vi "测验程序2.vi"() -> ()   [LabVIEW 2017]
uses:
  <vilib>/userdefined/High Color/IMAQdx.ctl
  <vilib>/Platform/TimedLoop/XDataNode/timing_clust.ctl
  <vilib>/Platform/TimedLoop/XDataNode/nitl_modes.ctl
  <vilib>/Platform/TimedLoop/XDataNode/wakeup.ctl
  <vilib>/myRIO/Common/Instrument Driver Framework/myRIO v1.0/UART/vis/myRIO v1.0 Close UART.vi
  <vilib>/FPGAPlugInAG/myRIO-1900/niLvFpga_Open_myRIO-1900.vi
  <vilib>/rvi/interface/common/dynamic/niFpgaDynamicAddResources.vi
  <vilib>/myRIO/Common/Instrument Driver Framework/Utilities/vis/FPGA Ref Manager.vi
  <vilib>/Utility/error.llb/Error Cluster From Error Code.vi
  <vilib>/myRIO/Common/Instrument Driver Framework/Utilities/vis/Ref Counter.vi
  <vilib>/rvi/errors/niLvFpgaAdjustHostInterfaceError.vi
  <vilib>/FPGAPlugInAG/Dynamic/niLvFpga_Close_Dynamic.vi
  <vilib>/myRIO/Common/Instrument Driver Framework/myRIO v1.0/myRIO v1.0 Reset FPGA.vi
  <vilib>/myRIO/Common/Instrument Driver Framework/myRIO v1.0/IRQ/vis/myRIO v1.0 IRQ Info FGV.vi
  <vilib>/myRIO/Common/Instrument Driver Framework/myRIO v1.0/IRQ/vis/myRIO v1.0 Timer IRQ Info FGV.vi
  <vilib>/myRIO/Common/Instrument Driver Framework/myRIO v1.0/IRQ/vis/myRIO v1.0 ISR Agent.vi
  <vilib>/Platform/TimedLoop/XDataNode/XDataNode.xnode
  <vilib>/rvi/interface/nirviOpenFPGA/nirviOpenFPGA.xnode
  <vilib>/rvi/interface/nirviReadWriteControl/nirviReadWriteControl.xnode
  <vilib>/rvi/interface/nirviCloseFPGA/nirviCloseFPGA.xnode
  <vilib>/Platform/TimedLoop/XDataNode/XDNodeRunTimeDep.lvlib
  <vilib>/myRIO/Instrument Drivers/Utilities/Utilities.lvlib
  NiFpgaLv.dll
  <vilib>/rvi/interface/Simulation/niFpgaSimulationCallBeginRW.vi
  <vilib>/vision/driver/NI_Vision_Acquisition_Software.lvlib
  <vilib>/vision/NI_Vision_Development_Module.lvlib
panel:
  in  "停止":bool
  out "Image Out":T1(plugin-control)
  out "数量":i32[](array[numeric])
  out "大小":dbl[](array[numeric])
  in  "保留图像？":bool
  in  "停止 2":bool
  out "货物类型":dbl
  in  "初始步态":u16
  in  "长度":i32=20000
  in  "开始":bool
  in  "思币得":i32=60
  out "QTI":bool
  out "当前步态":u16
  out "超声波":u32[](array[numeric])
  # "4小蓝"
  # "3小红"
  # "2大蓝"
  # "100000"
  # "1大红"
  # "70000"
  # "0异常"
  # "14600夹取高度"
  # "700夹住"
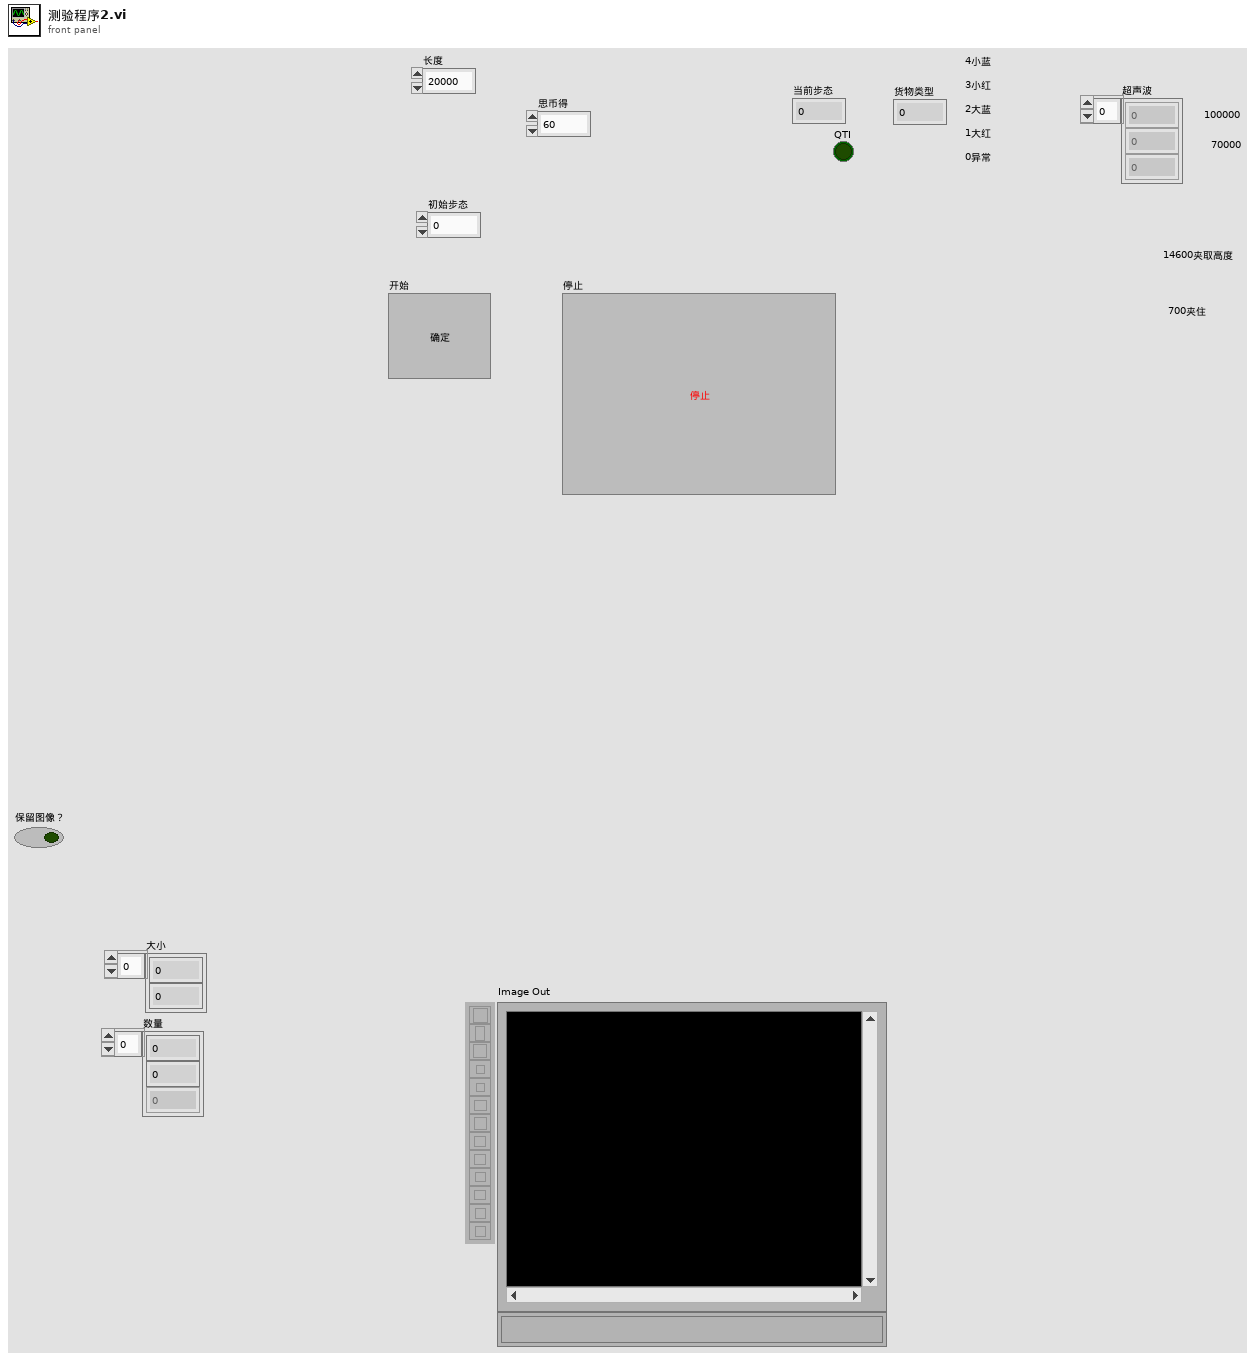
[diagram p1: front panel]
types:
  T1 = typedef "IMAQ Image.ctl" = refnum<image>
  T2 = typedef "IMAQdx.ctl" = refnum<k21>
  T3 = typedef "XDNodeRunTimeDep.lvlib/timing_clust.ctl" = cluster{"Expected End [f-1]":u64, "Actual End [f-1]":u64, "Finished Late? [f-1]":bool, "Expected End [i-1]":u64, "Actual End [i-1]":u64, "Finished Late? [i-1]":bool, "Expected Start [i]":u64, "Actual Start [i]":u64, "Expected Start [f]":u64, "Actual Start [f]":u64, "Source Name":string, "Structure Name":string, "Period":i64, "Deadline":i64, "Offset":i64, "Start":i64, "Priority":i32, "Timeout":i32, "Mode":T4, "Wakeup Reason":T5, "Error":errorcluster, "Source Type":string, "Secondary Source Type":string, "Global End Time":u64, "Global Start Time":u64, "Frame Duration":u64, "Iteration Duration":u64, "Assigned CPU":i32, "I/O Scan Engine Mode":u32}
  T4 = typedef "XDNodeRunTimeDep.lvlib/nitl_modes.ctl" = enum32{"No Change", "Process missed periods, maintain original phase", "Discard missed periods, maintain original phase", "Process missed periods, ignore original phase", "Discard missed periods, ignore original phase"}
  T5 = typedef "XDNodeRunTimeDep.lvlib/wakeup.ctl" = enum32{"Normal", "Aborted", "Asynchronous wakeup", "Timing source error", "Timed loop error", "Timeout"}
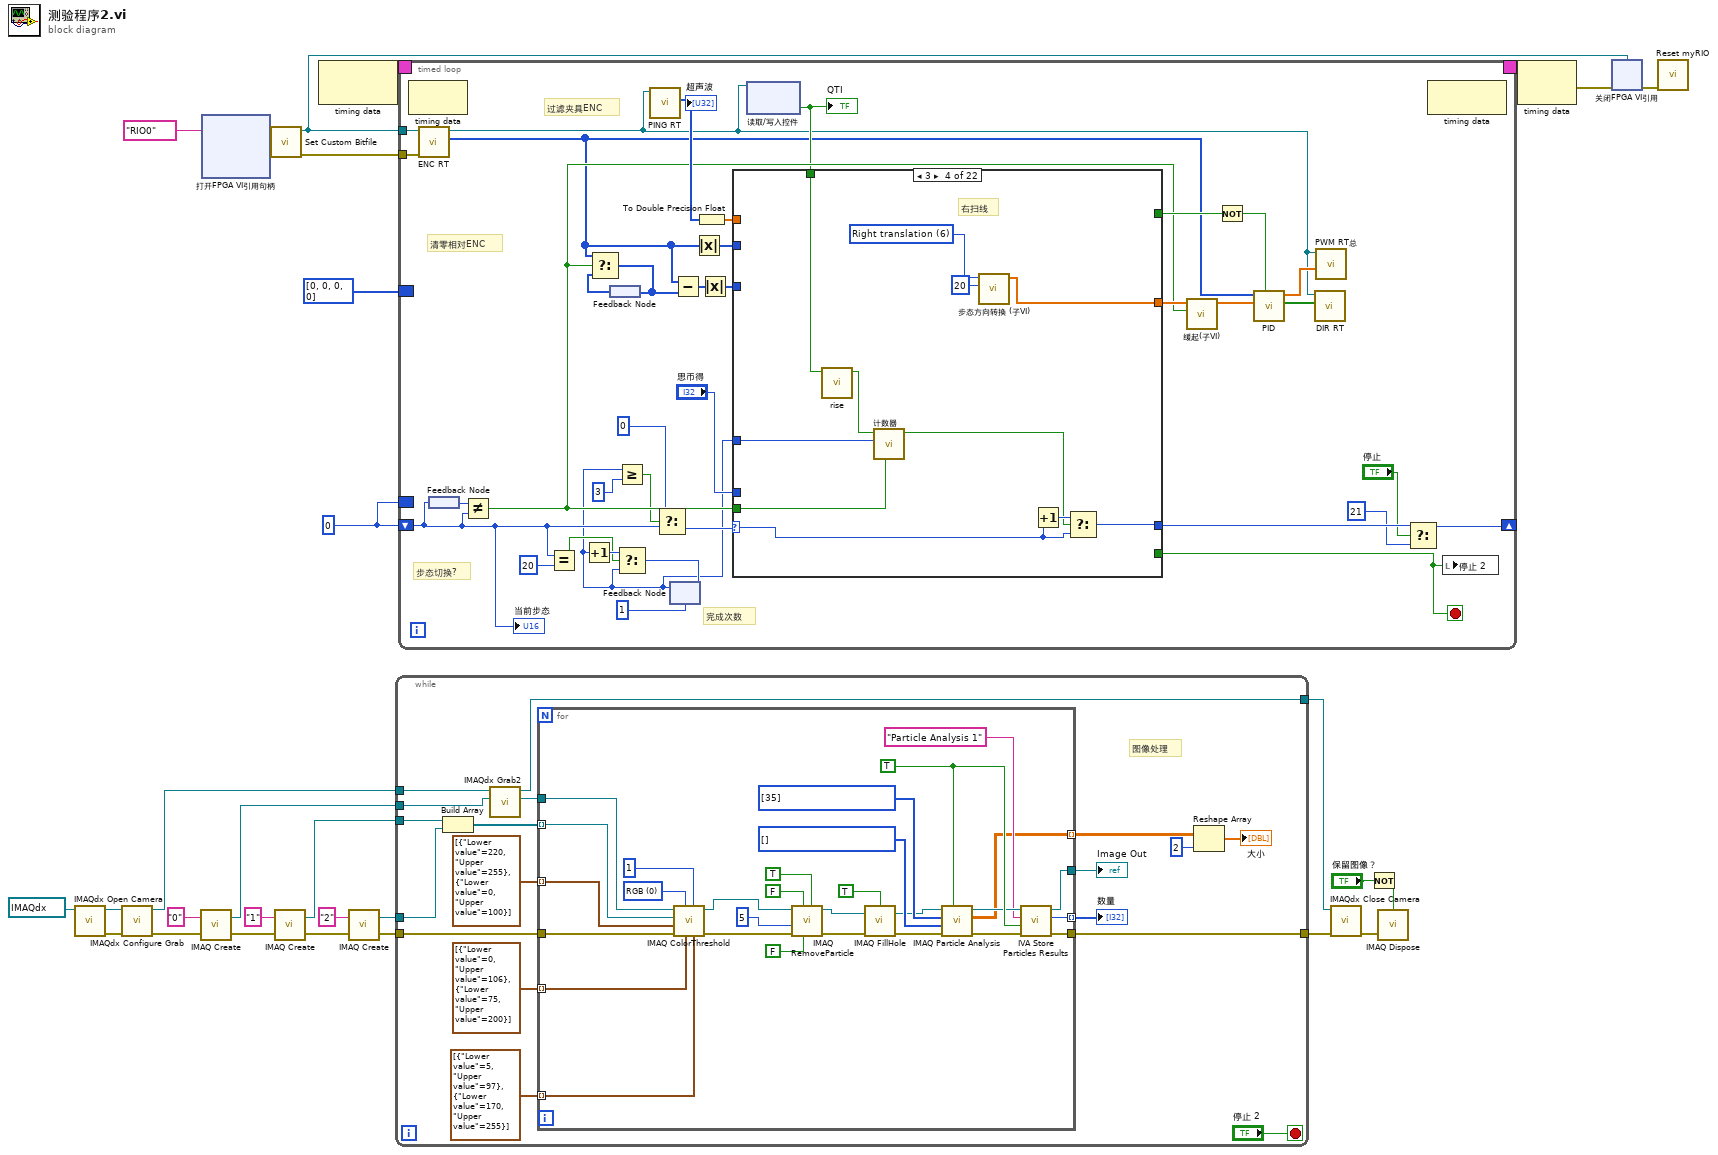
[diagram p0: block diagram]
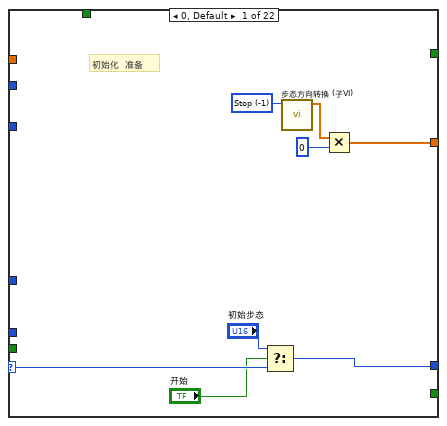
[diagram p2: hidden frame]
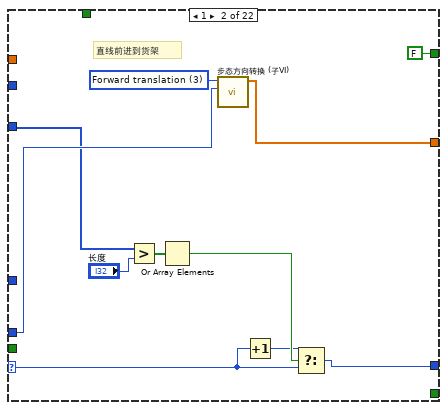
[diagram p3: hidden frame]
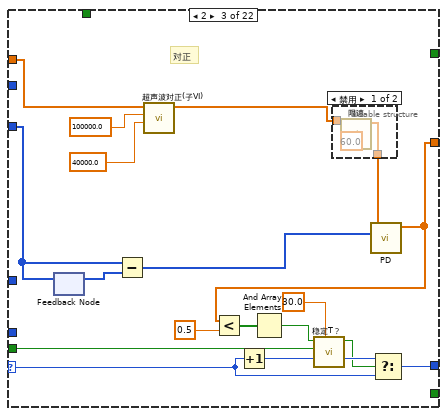
[diagram p4: hidden frame]
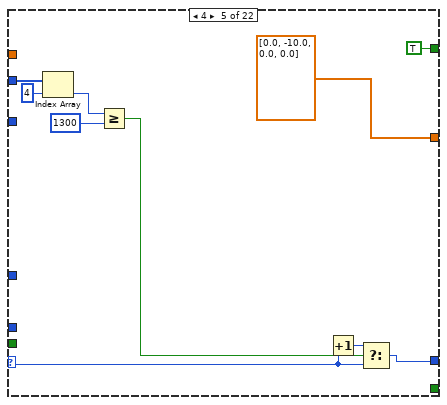
[diagram p6: hidden frame]
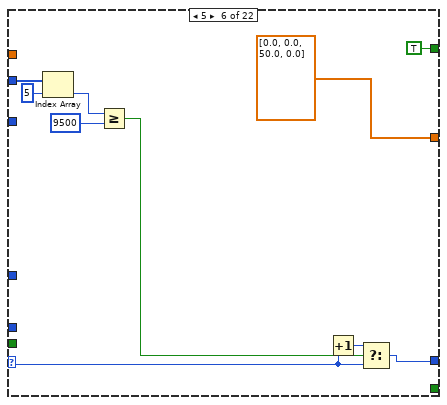
[diagram p7: hidden frame]
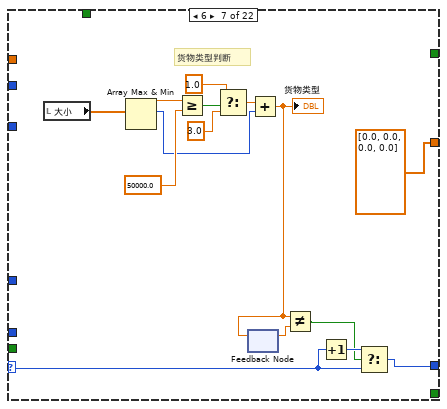
[diagram p8: hidden frame]
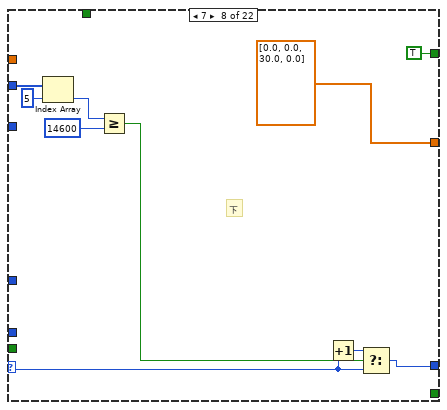
[diagram p9: hidden frame]
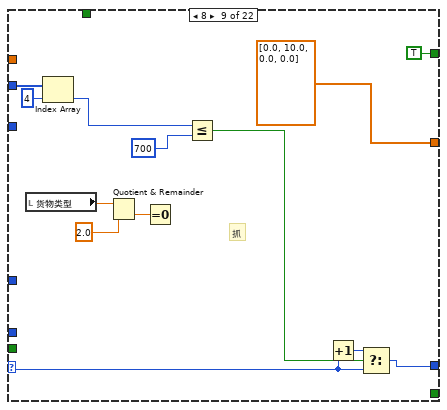
[diagram p10: hidden frame]
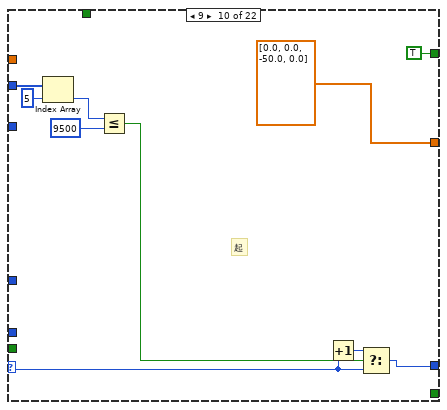
[diagram p11: hidden frame]
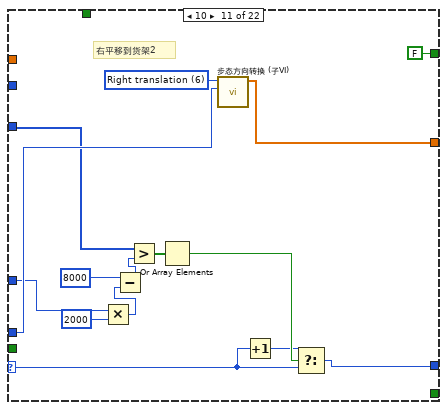
[diagram p12: hidden frame]
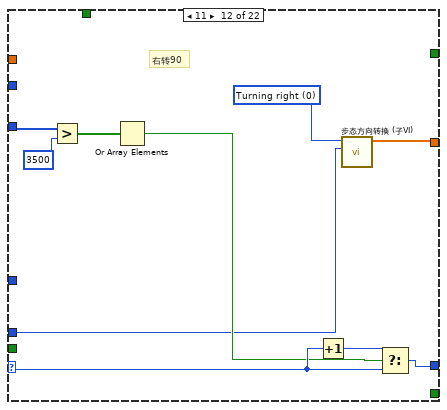
[diagram p13: hidden frame]
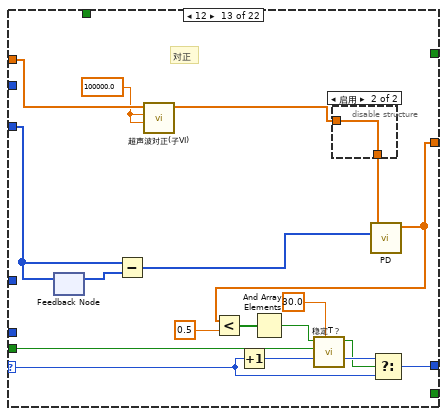
[diagram p14: hidden frame]
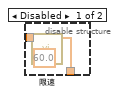
[diagram p15: hidden frame]
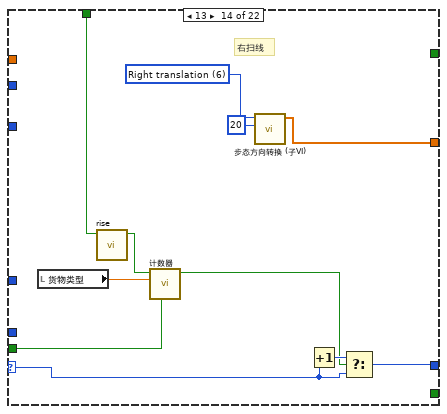
[diagram p16: hidden frame]
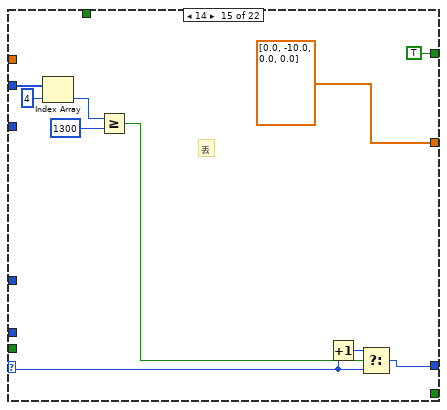
[diagram p17: hidden frame]
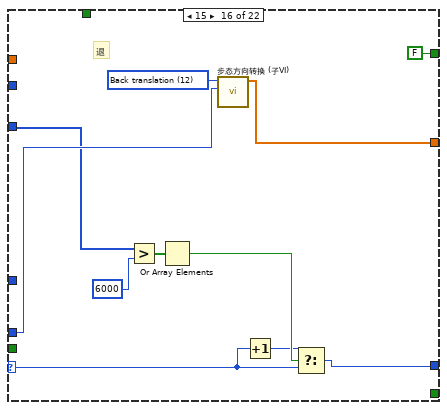
[diagram p18: hidden frame]
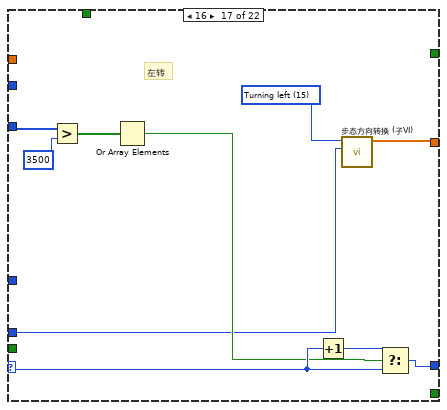
[diagram p19: hidden frame]
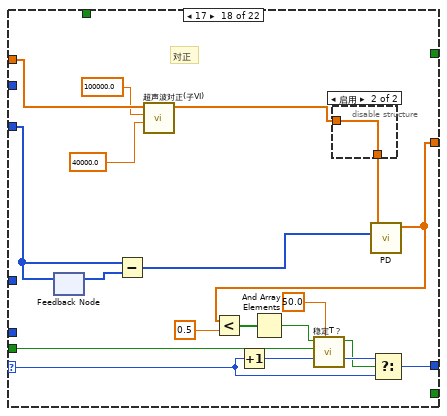
[diagram p20: hidden frame]
diagram:
  w28 = u16 0 ("初始步态")
  n1 = call <vilib>:"IMAQdx Open Camera.vi"("Session In"=T2 "cam0") -> ("error out"=w15:errorcluster, "Session Out"=w14:T2)  [unwired: 9 in]
  n2 = call <vilib>:"IMAQdx Configure Grab.vi"("error in"=w15, "Session In"=w14) -> ("error out"=w12:errorcluster, "Session Out"=w19:T2)  [unwired: 8 in]
  n3 = call "IMAQ Create"("Image Name"="0", "error in (no error)"=w12) -> ("New Image"=w17:T1, "error out"=w10:errorcluster)  [unwired: 3 in]
  n4 = xnode "打开FPGA VI引用句柄"("资源名称"=tag "RIO0") -> ("FPGA VI引用输出"=w24:refnum<k20>, "错误输出"=w23:errorcluster)  [unwired: 1 in]
  n5 = call <vilib>:"Set Custom Bitfile.vi"("error in (no error)"=w23, "Custom FPGA Reference In"=w24) -> ("error out"=w22:errorcluster, "Custom FPGA Reference Out"=w20:refnum<k20>)  [unwired: 8 in]
  n6 = call "IMAQ Create"("Image Name"="1", "error in (no error)"=w10) -> ("New Image"=w7:T1, "error out"=w8:errorcluster)  [unwired: 3 in]
  n7 = node-c288() -> (w30:T3)  [unwired: 1 in]
  n8 = call "IMAQ Create"("Image Name"="2", "error in (no error)"=w8) -> ("New Image"=w6:T1, "error out"=w5:errorcluster)  [unwired: 3 in]
  n9 = while {
    tunnel: w17 -> [w46]
    tunnel: w7 -> [w38]
    tunnel: w6 -> [w37]
    tunnel: w19 -> [w48]
    tunnel: [w47] -> w18
    tunnel: w5 -> [w33]
    tunnel: [w32] -> w4
    stop <- "停止 2" stop-if-true
    # "图像处理"
    n10 = Build Array(w38, w37) -> (w45:T1[])
    n11 = call <vilib>:"IMAQdx Grab2.vi"("Image In"=w46, "Session In"=w48) -> ("Image Out"=w39:T1, "Session Out"=w47:T2)  [unwired: 6 in, 2 out]
    n12 = for {
      tunnel: cluster{"Lower value":i32, "Upper value":i32}[] [{"Lower value"=220, "Upper value"=255}, {"Lower value"=0, "Upper value"=100}] -> [w75] mode=indexing
      tunnel: cluster{"Lower value":i32, "Upper value":i32}[] [{"Lower value"=0, "Upper value"=106}, {"Lower value"=75, "Upper value"=200}] -> [w74] mode=indexing
      tunnel: cluster{"Lower value":i32, "Upper value":i32}[] [{"Lower value"=5, "Upper value"=97}, {"Lower value"=170, "Upper value"=255}] -> [w73] mode=indexing
      tunnel: [w55] -> w40 mode=indexing
      tunnel: [w53] -> w36 mode=indexing
      tunnel: w39 -> [w52]
      tunnel: [w54] -> w44
      tunnel: w45 -> [w51] mode=indexing
      tunnel: w33 -> [w50]
      tunnel: [w49] -> w32
      w61 = i32[] [] items=["Center of Mass X", "Center of Mass Y", "First Pixel X", "First Pixel Y", "Bounding Rect Left", "Bounding Rect Top", "Bounding Rect Right", "Bounding Rect Bottom", "Max Feret Diameter Start X", "Max Feret Diameter Start Y", "Max Feret Diameter End X", "Max Feret Diameter End Y", "Max Horiz. Segment Length Left", "Max Horiz. Segment Length Right", "Max Horiz. Segment Length Row", "-", "Bounding Rect Width", "Bounding Rect Height", "Bounding Rect Diagonal", "Perimeter", "Convex Hull Perimeter", "Holes' Perimeter", "Max Feret Diameter", "Equivalent Ellipse Major Axis", "Equivalent Ellipse Minor Axis", "Equivalent Ellipse Minor Axis (Feret)", "Equivalent Rect Long Side", "Equivalent Rect Short Side", "Equivalent Rect Diagonal", "Equivalent Rect Short Side (Feret)", "Average Horiz. Segment Length", "Average Vert. Segment Length", "Hydraulic Radius", "Waddel Disk Diameter", "-", "Area", "Holes' Area", "Particle & Holes' Area", "Convex Hull Area", "Image Area", "-", "Number of Holes", "Number of Horiz. Segments", "Number of Vert. Segments", "-", "Orientation", "Max Feret Diameter Orientation", "-", "% Area/Image Area", "% Area/(Particle & Holes' Area)", "Ratio of Equivalent Ellipse Axes", "Ratio of Equivalent Rect Sides", "-", "Elongation Factor", "Compactness Factor", "Heywood Circularity Factor", "Type Factor", "-", "Sum X", "Sum Y", "Sum XX", "Sum XY", "Sum YY", "Sum XXX", "Sum XXY", "Sum XYY", "Sum YYY", "-", "Moment of Inertia XX", "Moment of Inertia XY", "Moment of Inertia YY", "Moment of Inertia XXX", "Moment of Inertia XXY", "Moment of Inertia XYY", "Moment of Inertia YYY", "Norm. Moment of Inertia XX", "Norm. Moment of Inertia XY", "Norm. Moment of Inertia YY", "Norm. Moment of Inertia XXX", "Norm. Moment of Inertia XXY", "Norm. Moment of Inertia XYY", "Norm. Moment of Inertia YYY", "Hu Moment 1", "Hu Moment 2", "Hu Moment 3", "Hu Moment 4", "Hu Moment 5", "Hu Moment 6", "Hu Moment 7"] ("Real-World Measurements")
      w62 = i32[] [35] items=["Center of Mass X", "Center of Mass Y", "First Pixel X", "First Pixel Y", "Bounding Rect Left", "Bounding Rect Top", "Bounding Rect Right", "Bounding Rect Bottom", "Max Feret Diameter Start X", "Max Feret Diameter Start Y", "Max Feret Diameter End X", "Max Feret Diameter End Y", "Max Horiz. Segment Length Left", "Max Horiz. Segment Length Right", "Max Horiz. Segment Length Row", "-", "Bounding Rect Width", "Bounding Rect Height", "Bounding Rect Diagonal", "Perimeter", "Convex Hull Perimeter", "Holes' Perimeter", "Max Feret Diameter", "Equivalent Ellipse Major Axis", "Equivalent Ellipse Minor Axis", "Equivalent Ellipse Minor Axis (Feret)", "Equivalent Rect Long Side", "Equivalent Rect Short Side", "Equivalent Rect Diagonal", "Equivalent Rect Short Side (Feret)", "Average Horiz. Segment Length", "Average Vert. Segment Length", "Hydraulic Radius", "Waddel Disk Diameter", "-", "Area", "Holes' Area", "Particle & Holes' Area", "Convex Hull Area", "Image Area", "-", "Number of Holes", "Number of Horiz. Segments", "Number of Vert. Segments", "-", "Orientation", "Max Feret Diameter Orientation", "-", "% Area/Image Area", "% Area/(Particle & Holes' Area)", "Ratio of Equivalent Ellipse Axes", "Ratio of Equivalent Rect Sides", "-", "Elongation Factor", "Compactness Factor", "Heywood Circularity Factor", "Type Factor", "-", "Sum X", "Sum Y", "Sum XX", "Sum XY", "Sum YY", "Sum XXX", "Sum XXY", "Sum XYY", "Sum YYY", "-", "Moment of Inertia XX", "Moment of Inertia XY", "Moment of Inertia YY", "Moment of Inertia XXX", "Moment of Inertia XXY", "Moment of Inertia XYY", "Moment of Inertia YYY", "Norm. Moment of Inertia XX", "Norm. Moment of Inertia XY", "Norm. Moment of Inertia YY", "Norm. Moment of Inertia XXX", "Norm. Moment of Inertia XXY", "Norm. Moment of Inertia XYY", "Norm. Moment of Inertia YYY", "Hu Moment 1", "Hu Moment 2", "Hu Moment 3", "Hu Moment 4", "Hu Moment 5", "Hu Moment 6", "Hu Moment 7"] ("Pixel Measurements")
      w59 = TRUE ("Connectivity 4/8 (8)")
      w76 = u16 0 items=["RGB", "HSL", "HSV", "HSI"] ("Color Mode")
      n13 = call "IMAQ ColorThreshold"("Blue or Luma or Val or Inten Range"=w73, "Replace Value"=1, "Green or Sat Range"=w74, "Color Mode"=w76, "error in (no error)"=w50, "Red or Hue Range"=w75, "Image Dst"=w51, "Image Src"=w52) -> ("error out"=w72:errorcluster, "Image Dst Out"=w67:T1)  [unwired: 2 out]
      n14 = call "IMAQ RemoveParticle"("Connectivity 4/8 (8)"=TRUE, "Low Pass/High Pass (Low)"=FALSE, "Square/Hexa (Square)"=FALSE, "error in (no error)"=w72, "Number of Erosion"=5, "Image Src"=w67) -> ("error out"=w66:errorcluster, "Image Dst Out"=w64:T1)  [unwired: 1 in, 3 out]
      n15 = call "IMAQ FillHole"("error in (no error)"=w66, "Image Src"=w64, "Connectivity 4/8 (8)"=TRUE) -> ("error out"=w63:errorcluster, "Image Dst Out"=w60:T1)  [unwired: 1 in, 2 out]
      n16 = call "IMAQ Particle Analysis"("Connectivity 4/8 (8)"=w59, "error in (no error)"=w63, "Real-World Measurements"=w61, "Pixel Measurements"=w62, "Image"=w60) -> ("error out"=w56:errorcluster, "Particle Measurements (Pixels)"=w53:dbl[][], "Image Out (duplicate)"=w58:T1)  [unwired: 4 out]
      n17 = call <vilib>:"IVA Store Particles Results.vi"("error in (no error)"=w56, "Connectivity 4/8 (8)"=w59, "Step Name"="Particle Analysis 1", "Image in"=w58) -> ("error out"=w49:errorcluster, "Number of Particles"=w55:i32, "Image dup"=w54:T1)  [unwired: 5 out]
    }
    "Image Out" <- w44
    "数量" <- w40
    n18 = Reshape Array(w36, 2 ("维数大小")) -> (→"大小":dbl[])
  }
  n19 = timed-loop {
    timing: w30 -> [_]
    timing-out: [_] -> w29
    shift-right: [w80] -> _
    shift-left: w28 -> [w89]
    border: w28 -> [_]
    border: i32[] [0, 0, 0, 0] ("ENC") -> [_]
    tunnel: w22 -> [w111]
    tunnel: w20 -> [w108]
    stop <- w81 stop-if-true
    # "完成次数"
    # "步态切换?"
    # "清零相对ENC"
    # "过滤夹具ENC"
    n20 = node-c288() -> ()  [unwired: 1 in, 1 out]
    n21 = call "ENC RT.vi"("错误输入（无错误）"=w111, "Custom FPGA Reference Out"=w108) -> ("ENC"=w96:i32[], "FPGA VI引用输出"=w94:refnum<k20>)  [unwired: 7 in, 1 out]
    n22 = feedback-in #1(w89) -> ()
    n23 = feedback #1() -> (w112:u16)
    n24 = Not Equal?(x=w112, y=w89) -> (x != y?=w99:bool)
    n25 = Equal?(x=w89, y=u16 20) -> (x = y?=w87:bool)
    n26 = feedback #2() -> (w110:i32[])
    n27 = Select(t=w96, s=w99, f=w110) -> (s? t:f=w93:i32[])
    n28 = feedback-in #2(w93) -> ()
    n29 = call "PING RT.vi"("引用句柄输入"=w94) -> ("PING"=w101:u32[])  [unwired: 8 in, 2 out]
    "超声波" <- w101
    n30 = feedback #3(1 ("次数")) -> (w82:i32)
    n31 = Increment(x=w82) -> (x+1=w91:i32)
    n32 = Greater Or Equal?(x=w82, y=3) -> (x >= y?=w83:bool)
    n33 = Select(t=w91, s=w87, f=w82) -> (s? t:f=w90:i32)
    n34 = Select(t=u16 0, s=w83, f=w89) -> (s? t:f=w86:u16)
    n35 = feedback-in #3(w90) -> ()
    n36 = Subtract(x=w96, y=w93) -> (x-y=w102:i32[])
    n37 = Absolute Value(x=w96) -> (abs(x)=w95:i32[])
    n38 = To Double Precision Float(number=w101) -> (double precision float=w100:dbl[])
    n39 = Absolute Value(x=w102) -> (abs(x)=w97:i32[])
    n40 = xnode "读取/写入控件"("FPGA VI引用输入"=w94) -> ("QTI"=w98:bool)  [unwired: 1 in, 2 out]
    "QTI" <- w98
    n41 = case shown="3" w86 {
      selector: w86 -> [w119 w125 w148 w163 w173 w183 w191 w208 w221 w231 w242 w252 w273 w288 w298 w304 w315 w337 w351 w361 _ w369]
      tunnel: [w120 w126 w142 w164 dbl[] [0.0, -10.0, 0.0, 0.0] ("输出") dbl[] [0.0, 0.0, 50.0, 0.0] ("输出") dbl[] [0.0, 0.0, 0.0, 0.0] ("输出") dbl[] [0.0, 0.0, 30.0, 0.0] ("输出") dbl[] [0.0, 10.0, 0.0, 0.0] ("输出") dbl[] [0.0, 0.0, -50.0, 0.0] ("输出") w243 w259 w267 w289 dbl[] [0.0, -10.0, 0.0, 0.0] ("输出") w305 w322 w331 dbl[] [0.0, 5.0, 0.0, 0.0] ("输出") dbl[] [0.0, 0.0, -40.0, 0.0] ("输出") dbl[] [0.0, 0.0, 0.0, 0.0] ("输出") dbl[] [0.0, 0.0, 0.0, 0.0] ("输出")] -> w107
      tunnel: "思币得" -> [_ w127 _ _ _ _ _ _ _ _ w244 w250 _ _ _ w306 w313 _ _ _ _ _]
      tunnel: [w117 w133 w147 w161 w175 w185 w193 w210 w223 w233 w249 w255 w272 w286 w300 w312 w318 w336 w353 w363 u16 2 ("初始步态") w369] -> w105
      tunnel: [_ FALSE ("继电器") _ _ TRUE ("继电器") TRUE ("继电器") _ TRUE ("继电器") TRUE ("继电器") TRUE ("继电器") FALSE ("继电器") _ _ _ TRUE ("继电器") FALSE ("继电器") _ _ TRUE ("继电器") TRUE ("继电器") _ _] -> w104
      tunnel: w97 -> [_ w123 w145 _ _ _ _ _ _ _ w240 w257 w270 _ _ w302 w320 w334 _ _ _ _]
      tunnel: w100 -> [_ _ w151 _ _ _ _ _ _ _ _ _ w276 _ _ _ _ w340 _ _ _ _]
      tunnel: w99 -> [_ _ w137 w157 _ _ _ _ _ _ _ _ w262 w282 _ _ _ w326 _ _ _ _]
      tunnel: w98 -> [_ _ _ w159 _ _ _ _ _ _ _ _ _ w284 _ _ _ _ _ _ _ _]
      tunnel: w95 -> [_ _ _ _ w167 w177 _ w202 w215 w225 _ _ _ _ w292 _ _ _ w345 w355 _ _]
      tunnel: w82 -> [_ _ _ w156 _ _ _ _ _ _ w239 _ _ _ _ _ _ _ _ _ _ _]
      tunnel: [_ _ _ _ _ _ _ _ _ _ _ _ _ _ _ _ _ _ _ _ _ TRUE ("停止 2")] -> w81
      frame 0, Default {
        w122 = i8 -1 items=["Stop"=-1, "Right translation"=6, "Back translation"=12, "Turning right"=0, "Turning left"=15, "Forward translation"=3, "Left translation"=9, "Gyro rotating"=16] ("Gait")
        # "初始化  准备"
        n42 = Select(t="初始步态", s="开始", f=w119) -> (s? t:f=w117:u16)
        n43 = call "步态方向转换 (子VI).vi"("Gait"=w122) -> ("输出"=w121:dbl[])  [unwired: 10 in]
        n44 = Multiply(x=w121, y=0 ("长度")) -> (x*y=w120:dbl[])
      }
      frame 1 {
        w128 = i8 3 items=["Stop"=-1, "Right translation"=6, "Back translation"=12, "Turning right"=0, "Turning left"=15, "Forward translation"=3, "Left translation"=9, "Gyro rotating"=16] ("Gait")
        # "直线前进到货架"
        n45 = Greater?(x=w123, y="长度") -> (0:w130:bool[])
        n46 = Or Array Elements(Boolean array=w130) -> (logical OR=w129:bool)
        n47 = call "步态方向转换 (子VI).vi"("速度"=w127, "Gait"=w128) -> ("输出"=w126:dbl[])  [unwired: 9 in]
        n48 = Increment(x=w125) -> (x+1=w124:u16)
        n49 = Select(t=w124, s=w129, f=w125) -> (s? t:f=w133:u16)
      }
      frame 2 {
        # "对正"
        n50 = feedback-in #4(w145) -> ()
        n51 = feedback #4() -> (w144:i32[])  [unwired: 1 in]
        n52 = Subtract(x=w145, y=w144) -> (x-y=w143:i32[])
        n53 = call "超声波对正(子VI).vi"("LFT"=40000.0, "FWD"=100000.0, "数组输入"=w151) -> ("数组输出"=w150:dbl[])  [unwired: 8 in]
        n54 = Increment(x=w148) -> (x+1=w149:u16)
        n55 = disable-structure shown="禁用" {
          disable-tunnel: w150 -> [w154 w155]
          disable-tunnel: [w152 w155] -> w146
          frame Disabled {
            n56 = call "限速.vi"("最大值"=60.0, "输入"=w154) -> ("数组"=w152:dbl[])  [unwired: 9 in]
          }
          frame Enabled {
          }
        }
        n57 = call "PD.vi"("ENC"=w143, "SET"=w146) -> ("output"=w142:dbl[])  [unwired: 9 in]
        n58 = Less?(x=w142, y=0.5) -> (x < y?=w140:bool[])
        n59 = And Array Elements(Boolean array=w140) -> (logical AND=w139:bool)
        n60 = call "稳定T？.vi"("次数(100)"=30.0, "Reset"=w137, "输入"=w139) -> ("TT？"=w138:bool)  [unwired: 8 in]
        n61 = Select(t=w149, s=w138, f=w148) -> (s? t:f=w147:u16)
      }
      frame 3 {
        w166 = i8 6 items=["Stop"=-1, "Right translation"=6, "Back translation"=12, "Turning right"=0, "Turning left"=15, "Forward translation"=3, "Left translation"=9, "Gyro rotating"=16] ("Gait")
        # "右扫线"
        n62 = call "rise.vi"("TF"=w159) -> ("UP?"=w158:bool)  [unwired: 10 in]
        n63 = call "计数器.vi"("Reset"=w157, "次数"=w156, "UP?"=w158) -> ("大于?"=w160:bool)  [unwired: 8 in]
        n64 = call "步态方向转换 (子VI).vi"("速度"=20, "Gait"=w166) -> ("输出"=w164:dbl[])  [unwired: 9 in]
        n65 = Increment(x=w163) -> (x+1=w162:u16)
        n66 = Select(t=w162, s=w160, f=w163) -> (s? t:f=w161:u16)
      }
      frame 4 {
        n67 = Index Array(array=w167, index=4 ("索引")) -> (element=w170:i32)
        n68 = Greater Or Equal?(x=w170, y=1300) -> (x >= y?=w168:bool)
        n69 = Increment(x=w173) -> (x+1=w174:u16)
        n70 = Select(t=w174, s=w168, f=w173) -> (s? t:f=w175:u16)
      }
      frame 5 {
        n71 = Index Array(array=w177, index=5 ("索引")) -> (element=w180:i32)
        n72 = Greater Or Equal?(x=w180, y=9500) -> (x >= y?=w178:bool)
        n73 = Increment(x=w183) -> (x+1=w184:u16)
        n74 = Select(t=w184, s=w178, f=w183) -> (s? t:f=w185:u16)
      }
      frame 6 {
        # "货物类型判断"
        n75 = local read "大小"() -> (w190:dbl[])
        n76 = Array Max & Min(array=w190) -> (max value=w200:dbl, max index (indices)=w195:i32)  [unwired: 2 out]
        n77 = Greater Or Equal?(x=w200, y=50000.0 ("大小阈值")) -> (x >= y?=w201:bool)
        n78 = Select(t=1.0, s=w201, f=3.0) -> (s? t:f=w196:dbl)
        n79 = feedback #5() -> (w189:dbl)  [unwired: 1 in]
        n80 = Add(x=w196, y=w195) -> (x+y=w188:dbl)
        "货物类型" <- w188
        n81 = feedback-in #5(w188) -> ()
        n82 = Not Equal?(x=w188, y=w189) -> (x != y?=w187:bool)
        n83 = Increment(x=w191) -> (x+1=w192:u16)
        n84 = Select(t=w192, s=w187, f=w191) -> (s? t:f=w193:u16)
      }
      frame 7 {
        # "下"
        n85 = Index Array(array=w202, index=5 ("索引")) -> (element=w205:i32)
        n86 = Greater Or Equal?(x=w205, y=14600) -> (x >= y?=w203:bool)
        n87 = Increment(x=w208) -> (x+1=w209:u16)
        n88 = Select(t=w209, s=w203, f=w208) -> (s? t:f=w210:u16)
      }
      frame 8 {
        # "抓"
        n89 = local read "货物类型"() -> (w214:dbl)
        n90 = Index Array(array=w215, index=4 ("索引")) -> (element=w218:i32)
        n91 = Quotient & Remainder(x=w214, y=2.0) -> (floor(x/y)=w212:dbl)  [unwired: 1 out]
        n92 = Equal To 0?(x=w212) -> ()  [unwired: 1 out]
        n93 = Less Or Equal?(x=w218, y=700) -> (x <= y?=w216:bool)
        n94 = Increment(x=w221) -> (x+1=w222:u16)
        n95 = Select(t=w222, s=w216, f=w221) -> (s? t:f=w223:u16)
      }
      frame 9 {
        # "起"
        n96 = Index Array(array=w225, index=5 ("索引")) -> (element=w228:i32)
        n97 = Less Or Equal?(x=w228, y=9500) -> (x <= y?=w226:bool)
        n98 = Increment(x=w231) -> (x+1=w232:u16)
        n99 = Select(t=w232, s=w226, f=w231) -> (s? t:f=w233:u16)
      }
      frame 10 {
        w245 = i8 6 items=["Stop"=-1, "Right translation"=6, "Back translation"=12, "Turning right"=0, "Turning left"=15, "Forward translation"=3, "Left translation"=9, "Gyro rotating"=16] ("Gait")
        # "右平移到货架2"
        n100 = Multiply(x=w239, y=2000) -> (x*y=w236:i32)
        n101 = Subtract(x=8000 ("长度 2"), y=w236) -> (x-y=w235:i32)
        n102 = Greater?(x=w240, y=w235) -> (0:w247:bool[])
        n103 = Or Array Elements(Boolean array=w247) -> (logical OR=w246:bool)
        n104 = call "步态方向转换 (子VI).vi"("速度"=w244, "Gait"=w245) -> ("输出"=w243:dbl[])  [unwired: 9 in]
        n105 = Increment(x=w242) -> (x+1=w241:u16)
        n106 = Select(t=w241, s=w246, f=w242) -> (s? t:f=w249:u16)
      }
      frame 11 {
        w258 = i8 0 items=["Stop"=-1, "Right translation"=6, "Back translation"=12, "Turning right"=0, "Turning left"=15, "Forward translation"=3, "Left translation"=9, "Gyro rotating"=16] ("Gait")
        # "右转90"
        n107 = Greater?(x=w257, y=3500) -> (0:w254:bool[])
        n108 = Or Array Elements(Boolean array=w254) -> (logical OR=w251:bool)
        n109 = Increment(x=w252) -> (x+1=w253:u16)
        n110 = call "步态方向转换 (子VI).vi"("速度"=w250, "Gait"=w258) -> ("输出"=w259:dbl[])  [unwired: 9 in]
        n111 = Select(t=w253, s=w251, f=w252) -> (s? t:f=w255:u16)
      }
      frame 12 {
        w260 = 100000.0 ("FWD")
        # "对正"
        n112 = feedback-in #6(w270) -> ()
        n113 = feedback #6() -> (w269:i32[])  [unwired: 1 in]
        n114 = Subtract(x=w270, y=w269) -> (x-y=w268:i32[])
        n115 = call "超声波对正(子VI).vi"("LFT"=w260, "FWD"=w260, "数组输入"=w276) -> ("数组输出"=w275:dbl[])  [unwired: 8 in]
        n116 = Increment(x=w273) -> (x+1=w274:u16)
        n117 = disable-structure shown="启用" {
          disable-tunnel: w275 -> [w279 w280]
          disable-tunnel: [w277 w280] -> w271
          frame Disabled {
            n118 = call "限速.vi"("最大值"=60.0, "输入"=w279) -> ("数组"=w277:dbl[])  [unwired: 9 in]
          }
          frame Enabled {
          }
        }
        n119 = call "PD.vi"("ENC"=w268, "SET"=w271) -> ("output"=w267:dbl[])  [unwired: 9 in]
        n120 = Less?(x=w267, y=0.5) -> (x < y?=w265:bool[])
        n121 = And Array Elements(Boolean array=w265) -> (logical AND=w264:bool)
        n122 = call "稳定T？.vi"("次数(100)"=30.0, "Reset"=w262, "输入"=w264) -> ("TT？"=w263:bool)  [unwired: 8 in]
        n123 = Select(t=w274, s=w263, f=w273) -> (s? t:f=w272:u16)
      }
      frame 13 {
        w291 = i8 6 items=["Stop"=-1, "Right translation"=6, "Back translation"=12, "Turning right"=0, "Turning left"=15, "Forward translation"=3, "Left translation"=9, "Gyro rotating"=16] ("Gait")
        # "右扫线"
        n124 = local read "货物类型"() -> (w281:dbl)
        n125 = call "rise.vi"("TF"=w284) -> ("UP?"=w283:bool)  [unwired: 10 in]
        n126 = call "计数器.vi"("Reset"=w282, "次数"=w281, "UP?"=w283) -> ("大于?"=w285:bool)  [unwired: 8 in]
        n127 = call "步态方向转换 (子VI).vi"("速度"=20, "Gait"=w291) -> ("输出"=w289:dbl[])  [unwired: 9 in]
        n128 = Increment(x=w288) -> (x+1=w287:u16)
        n129 = Select(t=w287, s=w285, f=w288) -> (s? t:f=w286:u16)
      }
      frame 14 {
        # "丢"
        n130 = Index Array(array=w292, index=4 ("索引")) -> (element=w295:i32)
        n131 = Greater Or Equal?(x=w295, y=1300) -> (x >= y?=w293:bool)
        n132 = Increment(x=w298) -> (x+1=w299:u16)
        n133 = Select(t=w299, s=w293, f=w298) -> (s? t:f=w300:u16)
      }
      frame 15 {
        w307 = i8 12 items=["Stop"=-1, "Right translation"=6, "Back translation"=12, "Turning right"=0, "Turning left"=15, "Forward translation"=3, "Left translation"=9, "Gyro rotating"=16] ("Gait")
        # "退"
        n134 = Greater?(x=w302, y=6000 ("长度 2")) -> (0:w309:bool[])
        n135 = Or Array Elements(Boolean array=w309) -> (logical OR=w308:bool)
        n136 = call "步态方向转换 (子VI).vi"("速度"=w306, "Gait"=w307) -> ("输出"=w305:dbl[])  [unwired: 9 in]
        n137 = Increment(x=w304) -> (x+1=w303:u16)
        n138 = Select(t=w303, s=w308, f=w304) -> (s? t:f=w312:u16)
      }
      frame 16 {
        w321 = i8 15 items=["Stop"=-1, "Right translation"=6, "Back translation"=12, "Turning right"=0, "Turning left"=15, "Forward translation"=3, "Left translation"=9, "Gyro rotating"=16] ("Gait")
        # "左转"
        n139 = Greater?(x=w320, y=3500) -> (0:w317:bool[])
        n140 = Or Array Elements(Boolean array=w317) -> (logical OR=w314:bool)
        n141 = Increment(x=w315) -> (x+1=w316:u16)
        n142 = call "步态方向转换 (子VI).vi"("速度"=w313, "Gait"=w321) -> ("输出"=w322:dbl[])  [unwired: 9 in]
        n143 = Select(t=w316, s=w314, f=w315) -> (s? t:f=w318:u16)
      }
      frame 17 {
        # "对正"
        n144 = feedback-in #7(w334) -> ()
        n145 = feedback #7() -> (w333:i32[])  [unwired: 1 in]
        n146 = Subtract(x=w334, y=w333) -> (x-y=w332:i32[])
        n147 = call "超声波对正(子VI).vi"("LFT"=40000.0, "FWD"=100000.0, "数组输入"=w340) -> ("数组输出"=w339:dbl[])  [unwired: 8 in]
        n148 = Increment(x=w337) -> (x+1=w338:u16)
        n149 = disable-structure shown="启用" {
          disable-tunnel: w339 -> [w343 w344]
          disable-tunnel: [w341 w344] -> w335
          frame Disabled {
            n150 = call "限速.vi"("最大值"=60.0, "输入"=w343) -> ("数组"=w341:dbl[])  [unwired: 9 in]
          }
          frame Enabled {
          }
        }
        n151 = call "PD.vi"("ENC"=w332, "SET"=w335) -> ("output"=w331:dbl[])  [unwired: 9 in]
        n152 = Less?(x=w331, y=0.5) -> (x < y?=w329:bool[])
        n153 = And Array Elements(Boolean array=w329) -> (logical AND=w328:bool)
        n154 = call "稳定T？.vi"("次数(100)"=50.0, "Reset"=w326, "输入"=w328) -> ("TT？"=w327:bool)  [unwired: 8 in]
        n155 = Select(t=w338, s=w327, f=w337) -> (s? t:f=w336:u16)
      }
      frame 18 {
        # "合手"
        n156 = Index Array(array=w345, index=4 ("索引")) -> (element=w348:i32)
        n157 = Less Or Equal?(x=w348, y=10) -> (x <= y?=w346:bool)
        n158 = Increment(x=w351) -> (x+1=w352:u16)
        n159 = Select(t=w352, s=w346, f=w351) -> (s? t:f=w353:u16)
      }
      frame 19 {
        # "起"
        n160 = Index Array(array=w355, index=5 ("索引")) -> (element=w358:i32)
        n161 = Less Or Equal?(x=w358, y=50) -> (x <= y?=w356:bool)
        n162 = Increment(x=w361) -> (x+1=w362:u16)
        n163 = Select(t=w362, s=w356, f=w361) -> (s? t:f=w363:u16)
      }
      frame 20 {
        # "完成"
        n164 = local write "货物类型"(0.0 ("货物类型")) -> ()
      }
      frame 21 {
        # "停止"
        n165 = local write "货物类型"(0.0 ("货物类型")) -> ()
      }
    }
    n166 = call "缓起(子VI).vi"("缓起清零"=w99, "输入"=w107) -> ("输出"=w109:dbl[])  [unwired: 9 in]
    n167 = Not(x=w104) -> (.not. x?=w103:bool)
    n168 = call "PID.vi"("继电器"=w103, "SET"=w109, "ENC"=w96) -> ("DIR"=w113:bool[], "PWM"=w114:dbl[])  [unwired: 7 in]
    n169 = call "DIR RT.vi"("DIR"=w113, "Custom FPGA Reference Out"=w94) -> ()  [unwired: 8 in, 2 out]
    n170 = call "PWM RT总.vi"("PWM"=w114, "Custom FPGA Reference Out"=w94) -> ()  [unwired: 8 in, 2 out]
    n171 = Select(t=w105, s="停止", f=u16 21) -> (s? t:f=w80:u16)
    n172 = node-c288() -> ()  [unwired: 1 in, 1 out]
    n173 = local write "停止 2"(w81) -> ()
    "当前步态" <- w89
  }
  n174 = call <vilib>:"IMAQdx Close Camera.vi"("error in"=w4, "Session In"=w18) -> ("error out"=w16:errorcluster)  [unwired: 9 in]
  n175 = Not(x="保留图像？") -> (.not. x?=w2:bool)
  n176 = call "IMAQ Dispose"("All Images? (No)"=w2, "error in (no error)"=w16) -> ()  [unwired: 4 in, 1 out]
  n177 = node-c288(w29) -> (w26:errorcluster)
  n178 = xnode "关闭FPGA VI引用"("FPGA VI引用输入"=w20, "错误输入"=w26) -> ("错误输出"=w25:errorcluster)
  n179 = call <vilib>:"Reset myRIO.vi"("error in (no error)"=w25) -> ()  [unwired: 10 in, 1 out]
